vi "SaveToDropBox-WaveformGraph.vi"(0 "WaveformGraph Refnum":refnum<vi>) -> ()   [LabVIEW 2009]
uses:
  <vilib>/Utility/sysdir.llb/System Directory Type.ctl
  <vilib>/Utility/file.llb/Write To Spreadsheet File (DBL).vi
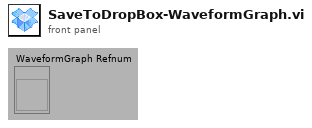
[diagram p1: front panel]
types:
  T1 = typedef "System Directory Type.ctl" = i32
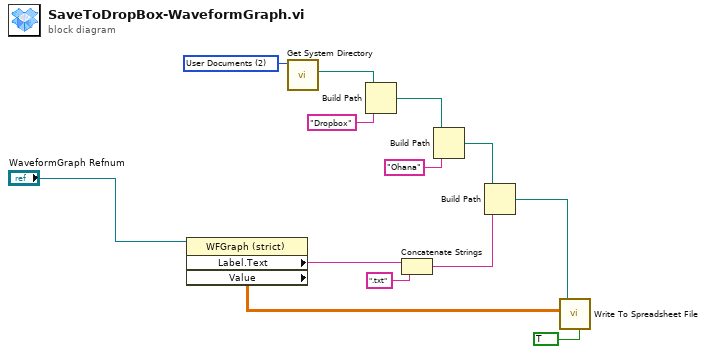
[diagram p0: block diagram]
diagram:
  w10 = T1 2 items=["User Home", "User Desktop", "User Documents", "User Application Data", "User Preferences", "User Temporary", "Public Documents", "Public Application Data", "Public Preferences", "System Core Libraries", "System Installed Libraries", "Application Files", "Boot Volume Root"] ("system directory type")
  n1 = property class="WFGraph (strict)"(reference="WaveformGraph Refnum") -> ("Label.Text"=w5:string, "Value"=w1:dbl[][])  [unwired: 1 in, 2 out]
  n2 = call <vilib>:"Get System Directory.vi"("system directory type"=w10) -> ("system directory"=w12:path)  [unwired: 10 in]
  n3 = Build Path(base path=w12, name or relative path="Dropbox") -> (appended path=w13:path)
  n4 = Concatenate Strings(w5, ".txt" ("string")) -> (w6:string)
  n5 = Build Path(base path=w13, name or relative path="Ohana") -> (appended path=w8:path)
  n6 = Build Path(base path=w8, name or relative path=w6) -> (appended path=w4:path)
  n7 = call-poly <vilib>:"Write To Spreadsheet File.vi"("transpose? (no:F)"=TRUE, "2D data"=w1, "file path (dialog if empty)"=w4) -> ()  [unwired: 5 in, 1 out]
